vi "WZ5005E-ONOFF.vi"(8 "error in":errorcluster caption="错误输入（无错误）", 9 "CMD":enum16{"输出OFF", "输出ON"}(ring), 10 "地址":string="02", 11 "MyIndex":u8) -> (0 "error out":errorcluster, 3 "Result":bool)   [LabVIEW 2015, in "WZ5005E.lvlib"]
uses:
  WZ5005E.lvlib
  <vilib>/Instr/_visa.llb/VISA Configure Serial Port (Instr).vi
panel:
  out "VISA":refnum<visa-resource-name>
  out "Send":string
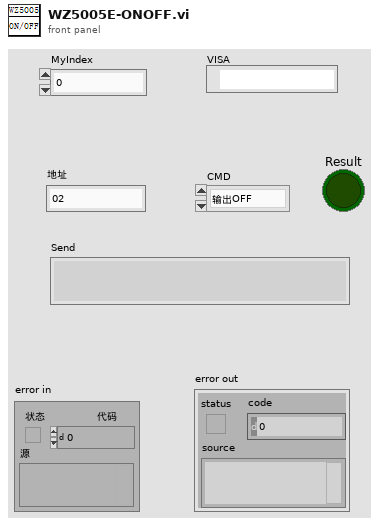
[diagram p1: front panel]
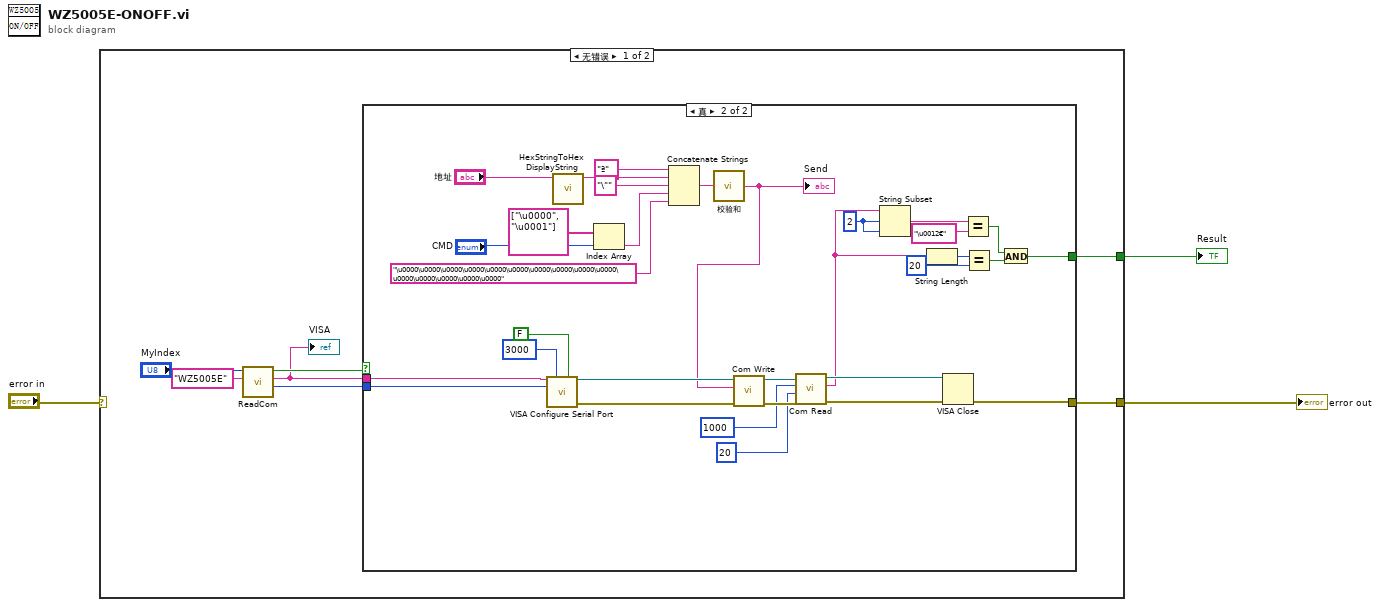
[diagram p0: block diagram]
diagram:
  n1 = case shown="无错误" "error in" {
    selector: "error in" -> [_ w43]
    tunnel: [w10 w43] -> w3
    tunnel: [w4 _] -> w1
    frame No Error {
      n2 = call "ReadCom.vi"("仪器名称"="WZ5005E", "MyIndex"="MyIndex") -> ("Baudrate"=w5:i32, "COM"=w6:string, "OK?"=w7:bool)  [unwired: 7 in]
      "VISA" <- w6
      n3 = case shown="真" w7 {
        tunnel: [_ w42] -> w10
        tunnel: w6 -> [_ w41]
        tunnel: w5 -> [_ w40]
        tunnel: [_ w12] -> w4
        frame False {
        }
        frame True {
          w19 = 2 ("偏移量(0)")
          n4 = call-poly "VISA Configure Serial Port"("VISA resource name"=w41, "timeout (10sec)"=u32 3000, "Enable Termination\nChar (T)"=FALSE ("Enable Termination\nChar (T)"), "baud rate (9600)"=w40) -> ("VISA resource name out"=w38:refnum<visa-resource-name>, "error out"=w37:errorcluster)  [unwired: 10 in]
          n5 = call "HexStringToHexDisplayString.vi"("正常显示HEX字符串"="地址") -> ("HEX显示字符串"=w24:string)  [unwired: 10 in]
          n6 = Index Array(array=string[] ["\u0000", "\u0001"], index="CMD") -> (element=w28:string)
          n7 = Concatenate Strings("ª", w24, "\"", w28, "\u0000\u0000\u0000\u0000\u0000\u0000\u0000\u0000\u0000\u0000\u0000\u0000\u0000\u0000\u0000") -> (w30:string)
          n8 = call "校验和.vi"("输入（Hex）"=w30) -> ("输出"=w21:string)
          "Send" <- w21
          n9 = call "Com Write.vi"("错误输入（无错误）"=w37, "Wbuff"=w21, "VISA In"=w38) -> ("错误输出"=w35:errorcluster, "VISA Out"=w36:refnum<visa-resource-name>)  [unwired: 6 in, 1 out]
          n10 = call "Com Read.vi"("错误输入（无错误）"=w35, "num"=u32 20, "超时"=u32 1000, "VISA In"=w36) -> ("错误输出"=w34:errorcluster, "buff"=w13:string, "VISA Out"=w33:refnum<visa-resource-name>)  [unwired: 4 in, 1 out]
          n11 = String Subset(string=w13, offset (0)=w19, length (rest)=w19) -> (substring=w18:string)
          n12 = String Length(string=w13) -> (length=w14:i32)
          n13 = VISA Close(VISA resource name=w33, error in (no error)=w34) -> (error out=w42:errorcluster)
          n14 = Equal?(x=w18, y="\u0012€" ("正则表达式")) -> (x = y?=w20:bool)
          n15 = Equal?(x=w14, y=20) -> (x = y?=w16:bool)
          n16 = And(x=w20, y=w16) -> (x .and. y?=w12:bool)
        }
      }
    }
    frame Error {
    }
  }
  "error out" <- w3
  "Result" <- w1
